vi "UART Configure Port.vi"(0 "UART Driver in":refnum<class "UART Driver.lvclass">, 1 "Port Number":u8, 5 "Baud":u32=4, 7 "Character Length":u8=8, 9 "Stop Bits":T1, 11 "error in":errorcluster, 12 "Parity":T2, 13 "Character Spacing (ticks)":u32=4) -> (4 "UART Driver out":refnum<class "UART Driver.lvclass">, 15 "error out":errorcluster)   [LabVIEW 2012, in "UART_Host_Driver.lvlib" / "UART Driver.lvclass"]
doc: "Initalize the UART port specificed by the RIO Device Name to the specified settings.\n\nMust call UART Initialize.vi, prior to calling UART Configure Port.vi.\n\nNote: Port Number 255 means to transmit to all of the ports configured in the UART Initialize.vi."
uses:
  UART Driver.lvclass
  FPGA/UART/Parity.ctl
  FPGA/UART/StopBits.ctl
  FPGA/UART/UART_Firmware.lvlib
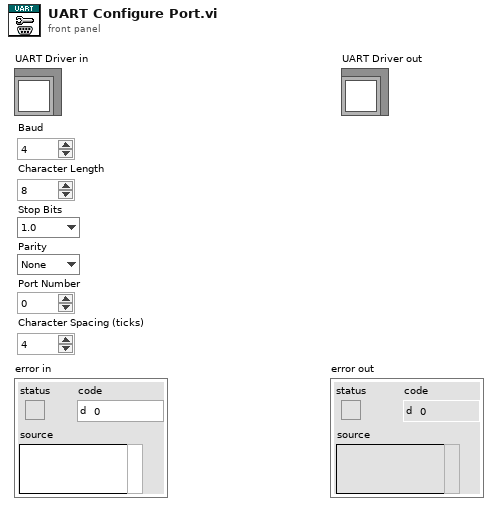
[diagram p1: front panel]
types:
  T1 = typedef "UART_Firmware.lvlib/StopBits.ctl" = enum8{"1.0", "1.5", "2.0"}
  T2 = typedef "UART_Firmware.lvlib/Parity.ctl" = enum8{"None", "Even", "Odd"}
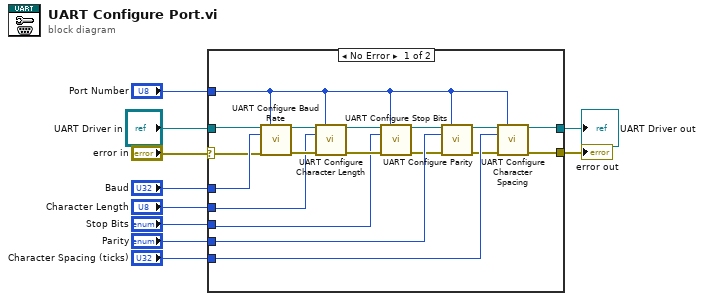
[diagram p0: block diagram]
diagram:
  n1 = case shown="No Error" "error in" {
    selector: "error in" -> [w26 w30]
    tunnel: [w11 w30] -> w9
    tunnel: [w15 w29] -> w2
    tunnel: "UART Driver in" -> [w28 w29]
    tunnel: "Baud" -> [w27 _]
    tunnel: "Character Length" -> [w23 _]
    tunnel: "Stop Bits" -> [w18 _]
    tunnel: "Parity" -> [w22 _]
    tunnel: "Port Number" -> [w14 _]
    tunnel: "Character Spacing (ticks)" -> [w13 _]
    frame No Error {
      n2 = call-dynamic "UART Configure Baud Rate.vi"("UART Driver in"=w28, "Port Number"=w14, "Baud Rate"=w27, "error in"=w26) -> ("UART Driver out"=w25:refnum<class "UART Driver.lvclass">, "error out"=w24:errorcluster)  [unwired: 9 in, 1 out]
      n3 = call-dynamic "UART Configure Character Length.vi"("UART Driver in"=w25, "Port Number"=w14, "Character Length"=w23, "error in"=w24) -> ("UART Driver out"=w20:refnum<class "UART Driver.lvclass">, "error out"=w19:errorcluster)  [unwired: 9 in, 1 out]
      n4 = call-dynamic "UART Configure Stop Bits.vi"("UART Driver in"=w20, "Port Number"=w14, "Stop Bits"=w18, "error in"=w19) -> ("UART Driver out"=w21:refnum<class "UART Driver.lvclass">, "error out"=w17:errorcluster)  [unwired: 9 in, 1 out]
      n5 = call-dynamic "UART Configure Parity.vi"("UART Driver in"=w21, "Channel Number"=w14, "Parity"=w22, "error in"=w17) -> ("UART Driver out"=w16:refnum<class "UART Driver.lvclass">, "error out"=w12:errorcluster)  [unwired: 9 in, 1 out]
      n6 = call-dynamic "UART Configure Character Spacing.vi"("UART Driver in"=w16, "Port Number"=w14, "Spacing (ticks)"=w13, "error in"=w12) -> ("UART Driver out"=w15:refnum<class "UART Driver.lvclass">, "error out"=w11:errorcluster)  [unwired: 9 in, 1 out]
    }
    frame Error {
    }
  }
  "error out" <- w9
  "UART Driver out" <- w2
